vi "Create.vi"(8 "error in (no error)":errorcluster) -> (0 "error out":errorcluster, 3 "Test Interface Mock Out":refnum<class "Test Interface Responsive Mock.lvclass">)   [LabVIEW 2020, in "Test Interface Responsive Mock.lvclass"]
uses:
  Test Interface Responsive Mock.lvclass
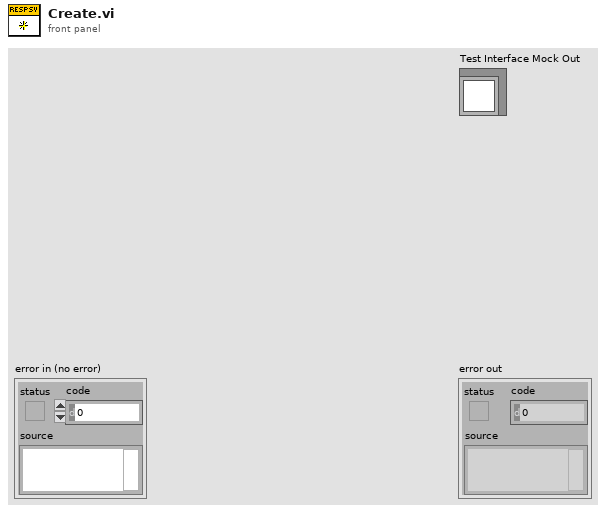
[diagram p1: front panel]
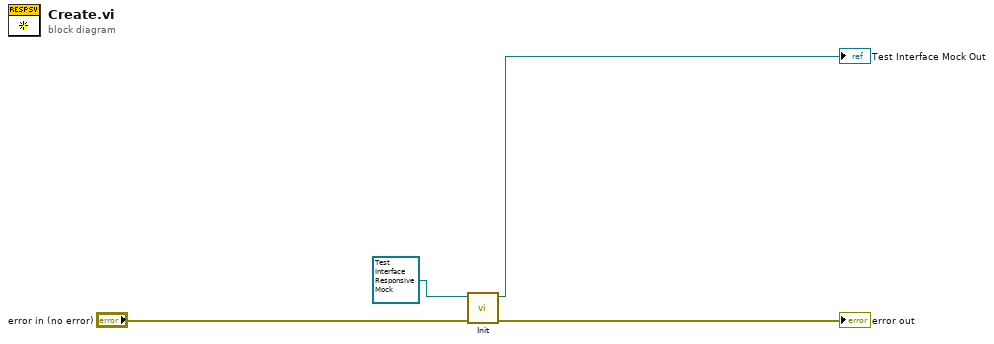
[diagram p0: block diagram]
diagram:
  n1 = call-dynamic "Init.vi"("error in (no error)"="error in (no error)", "Mock In"=refnum<class "Test Interface Responsive Mock.lvclass"> refnum ("Test Interface Mock.lvclass")) -> ("error out"=→"error out":errorcluster, "Mock Out"=→"Test Interface Mock Out":refnum<class "Test Interface Responsive Mock.lvclass">)  [unwired: 8 in]
